vi "dfd_Cascaded SOS Form II Normalization.vi"(7 "scale type":T1, 9 "coefficients b":dbl[](array[numeric]) format="%.2f", 10 "coefficients a":dbl[](array[numeric]) format="%.2f", 11 "x":dbl[](array[numeric])) -> (2 "norm":dbl[](array[numeric]) format="%.2f", 3 "y":dbl[](array[numeric]))   [LabVIEW 2017, in "NI_DigFilter_FXP.lvlib"]
uses:
  <vilib>/addons/Digital Filter Design/NI_DigFilter_FXP.lvlib
  <vilib>/addons/Digital Filter Design/_Objects.llb/DFD Coef Norm Type.ctl
  <vilib>/addons/Digital Filter Design/NI_DigFilterLicensed.lvlib
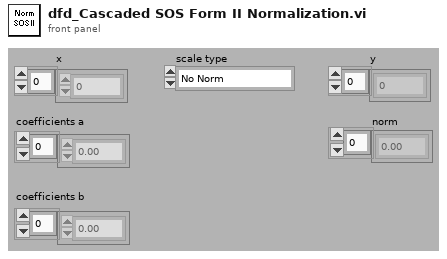
[diagram p1: front panel]
types:
  T1 = typedef "NI_DigFilterLicensed.lvlib/DFD Coef Norm Type.ctl" = enum16{"No Norm", "Time Domain 1-Norm", "Time Domain 2-Norm", "Time Domain Inf-Norm"}
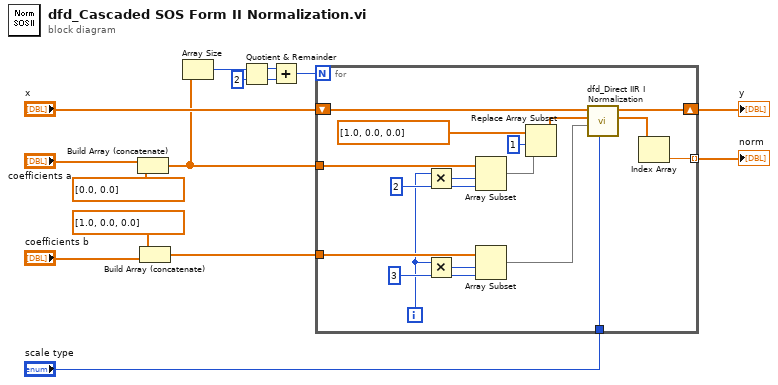
[diagram p0: block diagram]
diagram:
  n1 = Build Array (concatenate)("coefficients a", dbl[] [0.0, 0.0]) -> (w4:dbl[])
  n2 = Build Array (concatenate)(dbl[] [1.0, 0.0, 0.0], "coefficients b") -> (w1:dbl[])
  n3 = Array Size(array=w4) -> (size(s)=w12:i32)
  n4 = Quotient & Remainder(x=w12, y=2) -> (x-y*floor(x/y)=w14:i32, floor(x/y)=w13:i32)
  n5 = Add(x=w14, y=w13) -> (x+y=w11:i32)
  n6 = for {
    N: w11 -> [_]
    tunnel: w1 -> [w32]
    tunnel: w4 -> [w31]
    shift-right: [w19] -> w9
    shift-left: "x" -> [w25]
    tunnel: [w16] -> w7 mode=indexing
    tunnel: "scale type" -> [w18]
    i -> [w26]
    w28 = 2
    w30 = 3
    n7 = Multiply(x=w26, y=w28) -> (x*y=w27:i32)
    n8 = Multiply(x=w26, y=w30) -> (x*y=w29:i32)
    n9 = Array Subset(array=w31, index=w27, length=w28) -> (w22:dbl[])
    n10 = Array Subset(array=w32, index=w29, length=w30) -> (w24:dbl[])
    n11 = Replace Array Subset(array=dbl[] [1.0, 0.0, 0.0], new element=w22, index=1) -> (w20:dbl[])
    n12 = call <vilib>:"dfd_Direct IIR I Normalization.vi"("scale type"=w18, "coefficients b"=w24, "coefficients a"=w20, "x"=w25) -> ("norm"=w17:dbl[], "y"=w19:dbl[])  [unwired: 6 out]
    n13 = Index Array(array=w17) -> (element=w16:dbl)  [unwired: 1 in]
  }
  "norm" <- w7
  "y" <- w9
